vi "ID To Custom Device.vi"(8 "error in (no error)":errorcluster, 11 "ID in":T1 format="%.0x") -> (0 "error out":errorcluster, 2 "Device":refnum<k39>, 3 "ID out":u64 format="%.0x")   [LabVIEW 2026, in "Custom Devices Storage.lvlib"]
uses:
  Custom Devices Storage.lvlib
  <vilib>/NI VeriStand/Custom Device API/Custom Device Item Ref.ctl
  C:/Users/Administrator/Desktop/Jatin/All DNC DLLs/NationalInstruments.VeriStand.SystemDefinitionAPI.dll
  Jatin/All DNC DLLs/NationalInstruments.VeriStand.SystemDefinitionAPI.dll
  <vilib>/NI VeriStand/Custom Device API/Custom Device API.lvlib
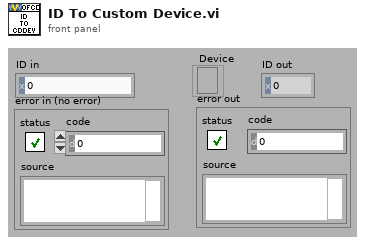
[diagram p1: front panel]
types:
  T1 = typedef "Custom Device API.lvlib/Custom Device Item Ref.ctl" = u64
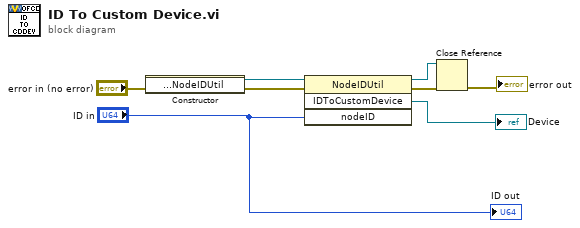
[diagram p0: block diagram]
diagram:
  n1 = constructor class="NodeIDUtil"(error in="error in (no error)") -> (reference out=w8:refnum<k39>, error out=w7:errorcluster)  [unwired: 2 in, 1 out]
  n2 = invoke class="NodeIDUtil" method="IDToCustomDevice"(reference=w8, error in=w7, "nodeID"="ID in") -> (reference out=w4:refnum<k39>, error out=w5:errorcluster, "IDToCustomDevice"=→"Device":refnum<k39>)  [unwired: 1 in, 1 out]
  n3 = Close Reference(reference=w4, error in (no error)=w5) -> (error out=→"error out":errorcluster)
  "ID out" <- "ID in"
